vi "MGI Bezier Fit Object.vi"(7 "Test Vector[]":dbl[](array[numeric]) format="%.2f", 8 "Substitution Matrix[][]":dbl[][](array[numeric]) format="%.2f", 9 "Constant Vector[]":dbl[](array[numeric]) format="%.2f", 10 "Sample Points[][]":dbl[][](array[numeric]) format="%.2f", 11 "Operation":T1) -> (0 "Log[][]":dbl[][](array[numeric]) format="%.2f", 1 "Bezier Points[][]":dbl[][](array[numeric]) format="%.2f", 2 "Model Curve":cluster{dbl[], dbl[]} {"?" format="%.2f"; "?" format="%.2f"}, 3 "Error":dbl format="%.2f")   [LabVIEW 2016]
doc: "Object used in fitting data to an n-dimensional Bezier curve. Sample points has n columns, m rows. Test vector is matrix multiplied by the substitution matrix and added to the constant vector, then the result is reshaped to n x 4. Bezier curve is sampled at m points for comparison to the sample points. Error is sum of squared distances between sample points and nearest points on the Bezier curve as sampled.\n\nAuthored by David A. Moore\nsupport@mooregoodideas.com\nwww.mooregoodideas.com\n\nCopyright (c) 2010, Moore Good Ideas, Inc.\n\nAll rights reserved.\n\nRedistribution and use in source and binary forms, with or without modification, are permitted provided that the following conditions are met:\n\n * Redistributions of source code must retain the above copyright notice, this list of conditions and the following disclaimer.\n * Redistributions in binary form must reproduce the above copyright notice, this list of conditions and the following disclaimer in the documentation and/or other materials provided with the distribution.\n * Neither the name of Moore Good Ideas, Inc. nor the names of its contributors may be used to endorse or promote products derived from this software without specific prior written permission.\n\nTHIS SOFTWARE IS PROVIDED BY THE COPYRIGHT HOLDERS AND CONTRIBUTORS \"AS IS\" AND ANY EXPRESS OR IMPLIED WARRANTIES, INCLUDING, BUT NOT LIMITED TO, THE IMPLIED WARRANTIES OF MERCHANTABILITY AND FITNESS FOR A PARTICULAR PURPOSE ARE DISCLAIMED. IN NO EVENT SHALL THE COPYRIGHT OWNER OR CONTRIBUTORS BE LIABLE FOR ANY DIRECT, INDIRECT, INCIDENTAL, SPECIAL, EXEMPLARY, OR CONSEQUENTIAL DAMAGES (INCLUDING, BUT NOT LIMITED TO, PROCUREMENT OF SUBSTITUTE GOODS OR SERVICES; LOSS OF USE, DATA, OR PROFITS; OR BUSINESS INTERRUPTION) HOWEVER CAUSED AND ON ANY THEORY OF LIABILITY, WHETHER IN CONTRACT, STRICT LIABILITY, OR TORT (INCLUDING NEGLIGENCE OR OTHERWISE) ARISING IN ANY WAY OUT OF THE USE OF THIS SOFTWARE, EVEN IF ADVISED OF THE POSSIBILITY OF SUCH DAMAGE."
uses:
  <userlib>/_MGI/Bezier/MGI Bezier Fit Operation Enumeration.ctl
  <vilib>/Analysis/baseanly.llb/A x Vector.vi
  <userlib>/_MGI/Bezier/MGI Bezier Vector/MGI Bezier Vector (DBL).vi
  <vilib>/Analysis/NI_AALBase.lvlib
panel:
  out "Output Array[][]":dbl[][](array[numeric]) format="%.2f"
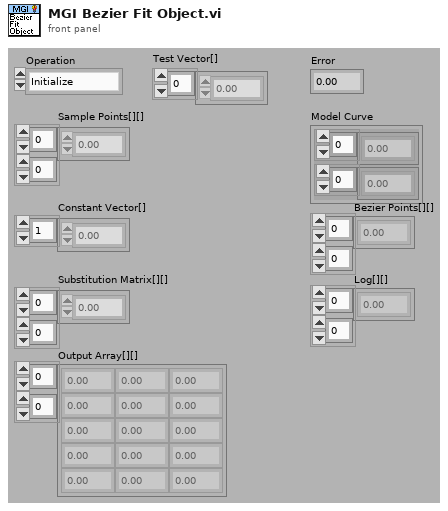
[diagram p1: front panel]
types:
  T1 = typedef "MGI Bezier Fit Operation Enumeration.ctl" = enum16{"Initialize", "Test", "Read Curve", "Calc Bezier Points"}
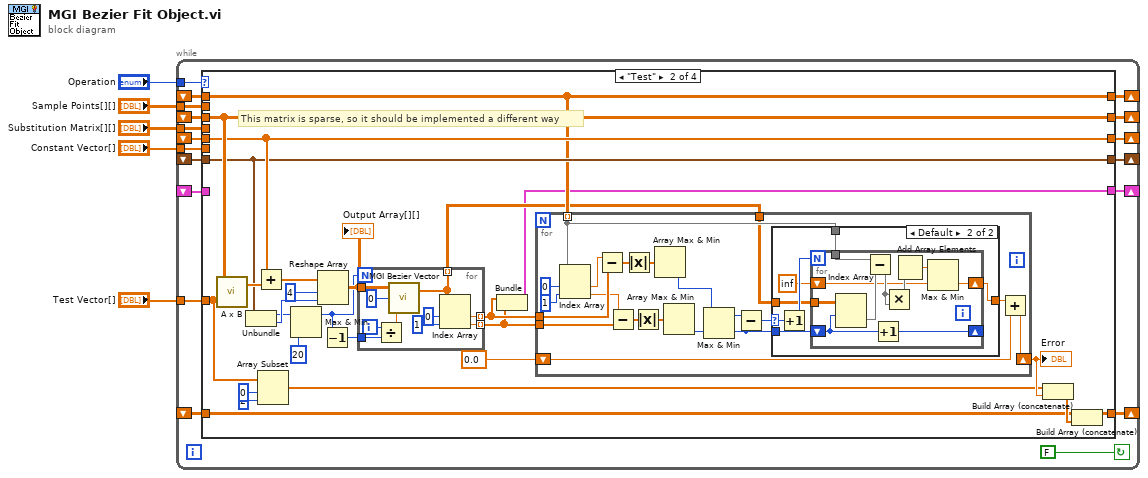
[diagram p0: block diagram]
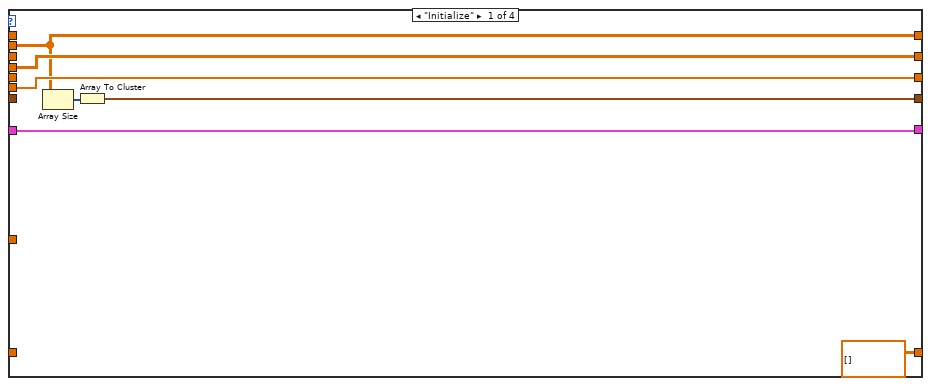
[diagram p2: hidden frame]
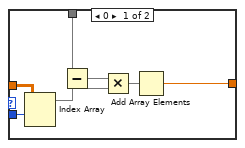
[diagram p3: hidden frame]
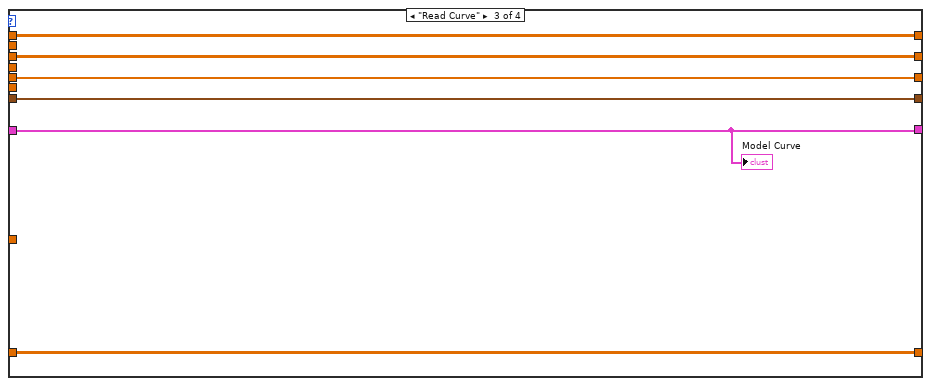
[diagram p4: hidden frame]
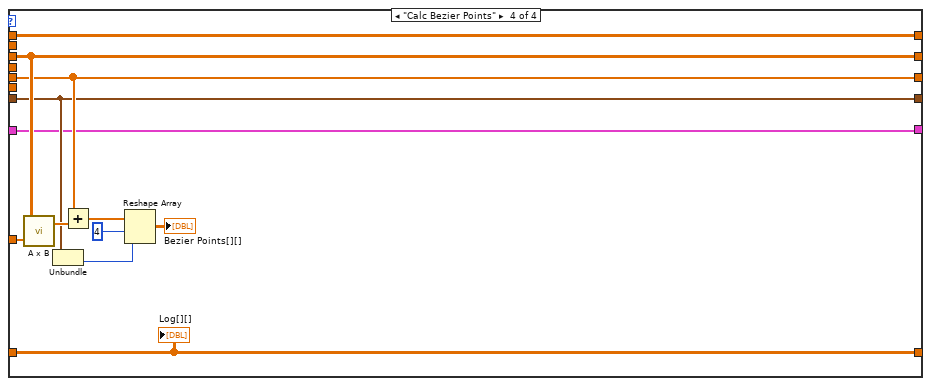
[diagram p5: hidden frame]
diagram:
  n1 = while {
    shift-left: _ -> [w6]
    shift-right: [w7] -> _
    shift-left: _ -> [w8]
    shift-right: [w9] -> _
    tunnel: "Test Vector[]" -> [w10]
    tunnel: "Constant Vector[]" -> [w17]
    tunnel: "Substitution Matrix[][]" -> [w18]
    tunnel: "Sample Points[][]" -> [w21]
    shift-left: _ -> [w11]
    shift-right: [w15] -> _
    shift-left: _ -> [w12]
    shift-right: [w16] -> _
    shift-left: _ -> [w13]
    shift-right: [w19] -> _
    shift-left: _ -> [w14]
    shift-right: [w20] -> _
    tunnel: "Operation" -> [w22]
    stop <- FALSE continue-if-true
    n2 = case shown="\"Test\"" w22 {
      tunnel: w21 -> [w28 _ _ _]
      tunnel: [w28 w48 w116 w120] -> w20
      tunnel: [w30 w56 w115 w127] -> w19
      tunnel: w18 -> [w30 _ _ _]
      tunnel: w17 -> [w29 _ _ _]
      tunnel: [w29 w54 w114 w125] -> w16
      tunnel: [w26 w52 w113 w123] -> w15
      tunnel: w14 -> [_ w48 w116 w120]
      tunnel: w13 -> [_ w56 w115 w127]
      tunnel: w12 -> [_ w54 w114 w125]
      tunnel: w11 -> [_ w52 w113 w123]
      tunnel: w10 -> [_ w39 _ w128]
      tunnel: [w25 w43 w112 w118] -> w9
      tunnel: w8 -> [w25 _ w112 w118]
      tunnel: [dbl[][] [] w35 w111 w117] -> w7
      tunnel: w6 -> [_ w34 w111 w117]
      frame "Initialize" {
        n3 = Array Size(array=w28) -> (size(s)=w27:i32[])
        n4 = Array To Cluster(array=w27) -> (cluster=w26:cluster{"[0]":i32, "[1]":i32})
      }
      frame "Test" {
        # "This matrix is sparse, so it should be implemented a different way"
        n5 = call-poly <vilib>:"A x B.vi"("Vector"=w39, "A"=w56) -> ("A x Vector"=w55:dbl[])  [unwired: 1 out]
        n6 = Unbundle(w52) -> ("[0]"=w33:i32, "[1]"=w50:i32)
        n7 = Add(x=w54, y=w55) -> (x+y=w53:dbl[])
        n8 = Array Subset(array=w39, index=0 ("Array Index"), length=2 ("Array Length")) -> (w40:dbl[])
        n9 = Max & Min(x=w33, y=20) -> (max(x,y)=w32:i32)  [unwired: 1 out]
        n10 = Reshape Array(w53, 4 ("Dimension Size"), w50) -> (w42:dbl[][])
        "Output Array[][]" <- w42
        n11 = Decrement(x=w32) -> (x-1=w49:i32)
        n12 = for {
          N: w32 -> [_]
          tunnel: w42 -> [w110]
          tunnel: w49 -> [w107]
          tunnel: [w105] -> w46 mode=indexing
          tunnel: [w101] -> w45 mode=indexing
          tunnel: [w102] -> w44 mode=indexing
          i -> [w108]
          n13 = Divide(x=w108, y=w107) -> (x/y=w106:dbl)
          n14 = call-poly <userlib>:"MGI Bezier Vector.vi"("u"=w106, "First k"=0, "Bezier Control Points[k][dims]"=w110) -> ("N-dimensional Vector[]"=w105:dbl[])  [unwired: 1 out]
          n15 = Index Array(array=w105, index #1=0 ("Index"), index #2=1 ("Index")) -> (element #1=w101:dbl, element #2=w102:dbl)
        }
        n16 = Bundle(w45, w44) -> (w43:cluster{dbl[], dbl[]})  [unwired: 1 in]
        n17 = for {
          tunnel: w48 -> [w76] mode=indexing
          tunnel: w45 -> [w72]
          tunnel: w44 -> [w68]
          tunnel: w46 -> [w60]
          shift-right: [w59] -> w41
          shift-left: 0.0 -> [w57]
          n18 = Index Array(array=w76, index #1=0 ("Index"), index #2=1 ("Index")) -> (element #1=w73:dbl, element #2=w69:dbl)
          n19 = Subtract(x=w73, y=w72) -> (x-y=w71:dbl[])
          n20 = Subtract(x=w69, y=w68) -> (x-y=w67:dbl[])
          n21 = Absolute Value(x=w71) -> (abs(x)=w70:dbl[])
          n22 = Absolute Value(x=w67) -> (abs(x)=w66:dbl[])
          n23 = Array Max & Min(array=w70) -> (min index (indices)=w64:i32)  [unwired: 3 out]
          n24 = Array Max & Min(array=w66) -> (min index (indices)=w65:i32)  [unwired: 3 out]
          n25 = Max & Min(x=w64, y=w65) -> (max(x,y)=w63:i32, min(x,y)=w61:i32)
          n26 = Subtract(x=w63, y=w61) -> (x-y=w62:i32)
          n27 = case shown="Default" w62 {
            selector: w62 -> [_ w90]
            tunnel: w61 -> [w83 w89]
            tunnel: w60 -> [w82 w87]
            tunnel: w76 -> [w80 w86]
            tunnel: [w77 w84] -> w58
            frame 0 {
              n28 = Index Array(array=w82, index (row)=w83) -> (element=w81:dbl[])  [unwired: 1 in]
              n29 = Subtract(x=w80, y=w81) -> (x-y=w79:dbl[])
              n30 = Multiply(x=w79, y=w79) -> (x*y=w78:dbl[])
              n31 = Add Array Elements(numeric array=w78) -> (sum=w77:dbl)
            }
            frame Default {
              n32 = Increment(x=w90) -> (x+1=w88:i32)
              n33 = for {
                N: w88 -> [_]
                shift-right: [w100] -> _
                shift-left: w89 -> [w99]
                tunnel: w87 -> [w98]
                tunnel: w86 -> [w96]
                shift-right: [w93] -> w84
                shift-left: inf -> [w92]
                n34 = Index Array(array=w98, index (row)=w99) -> (element=w97:dbl[])  [unwired: 1 in]
                n35 = Subtract(x=w96, y=w97) -> (x-y=w95:dbl[])
                n36 = Increment(x=w99) -> (x+1=w100:i32)
                n37 = Multiply(x=w95, y=w95) -> (x*y=w94:dbl[])
                n38 = Add Array Elements(numeric array=w94) -> (sum=w91:dbl)
                n39 = Max & Min(x=w91, y=w92) -> (min(x,y)=w93:dbl)  [unwired: 1 out]
              }
            }
          }
          n40 = Add(x=w58, y=w57) -> (x+y=w59:dbl)
        }
        "Error" <- w41
        n41 = Build Array (concatenate)(w40, w41) -> (w36:dbl[])
        n42 = Build Array (concatenate)(w34, w36) -> (w35:dbl[][])
      }
      frame "Read Curve" {
        "Model Curve" <- w112
      }
      frame "Calc Bezier Points" {
        n43 = call-poly <vilib>:"A x B.vi"("Vector"=w128, "A"=w127) -> ("A x Vector"=w126:dbl[])  [unwired: 1 out]
        n44 = Unbundle(w123) -> ("[1]"=w121:i32)  [unwired: 1 out]
        n45 = Add(x=w125, y=w126) -> (x+y=w124:dbl[])
        n46 = Reshape Array(w124, 4 ("Dimension Size"), w121) -> (→"Bezier Points[][]":dbl[][])
        "Log[][]" <- w117
      }
    }
  }
